vi "ActionOnSegment.vi"(8 "error in (no error)":errorcluster, 10 "Path":path, 11 "Channel Manager in":refnum<class "Channel Manager.lvclass">) -> (0 "error out":errorcluster, 3 "Channel Manager out":refnum<class "Channel Manager.lvclass">)   [LabVIEW 2024, in "Embedded TDMS Logger Engine.lvlib" / "Channel Manager.lvclass"]
uses:
  Channel Manager.lvclass
  Channel Manager.lvclass/Channel Manager.ctl
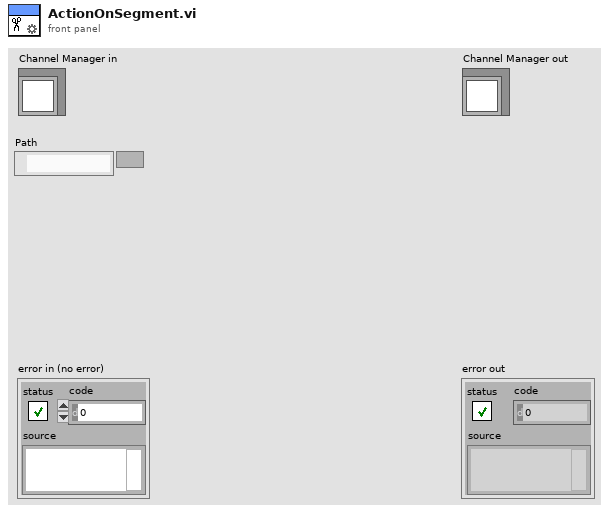
[diagram p1: front panel]
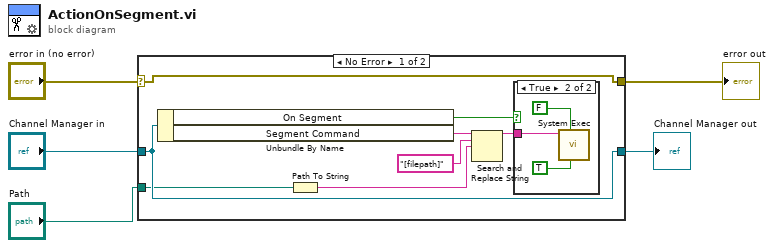
[diagram p0: block diagram]
diagram:
  n1 = case shown="No Error" "error in (no error)" {
    selector: "error in (no error)" -> [w13 w18]
    tunnel: [w13 w18] -> w4
    tunnel: [w11 w17] -> w2
    tunnel: "Channel Manager in" -> [w11 w17]
    tunnel: "Path" -> [w8 _]
    frame No Error {
      n2 = Unbundle By Name(w11) -> ("On Segment"=w12:bool, "Segment Command"=w10:string)
      n3 = Path To String(path=w8) -> (string=w7:string)
      n4 = Search and Replace String(input string=w10, search string="[filepath]", replace string=w7) -> (result string=w9:string)  [unwired: 5 in, 3 out]
      n5 = case shown="True" w12 {
        tunnel: w9 -> [_ w14]
        frame False {
        }
        frame True {
          n6 = call <vilib>:"System Exec.vi"("run minimized? (F)"=TRUE, "wait until completion? (T)"=FALSE, "command line"=w14) -> ()  [unwired: 5 in, 4 out]
        }
      }
    }
    frame Error {
    }
  }
  "error out" <- w4
  "Channel Manager out" <- w2
